vi "ProdaNG.Configurator.Glb.Read.vi"(7 "DB":T2, 8 "error in (no error)":errorcluster) -> (0 "error out":errorcluster, 1 "Configuration":T1={"ShowUnreleased"=TRUE, "Param1"="StepIndex", "ParamStartIdx"=0, "Slots"=1} {"Slots" min=1 max=2; "ParamStartIdx" min=0 max=1}, 2 "Data found":bool)   [LabVIEW 2016]
uses:
  ProdaNG.Configurator.DB.ctl
  ProdaNG.Configurator.Config.ctl
  Tools/Tma.lib/nlconfig.llb/fp2ini mode.ctl
  ProdaNG.Configurator.Glb.vi
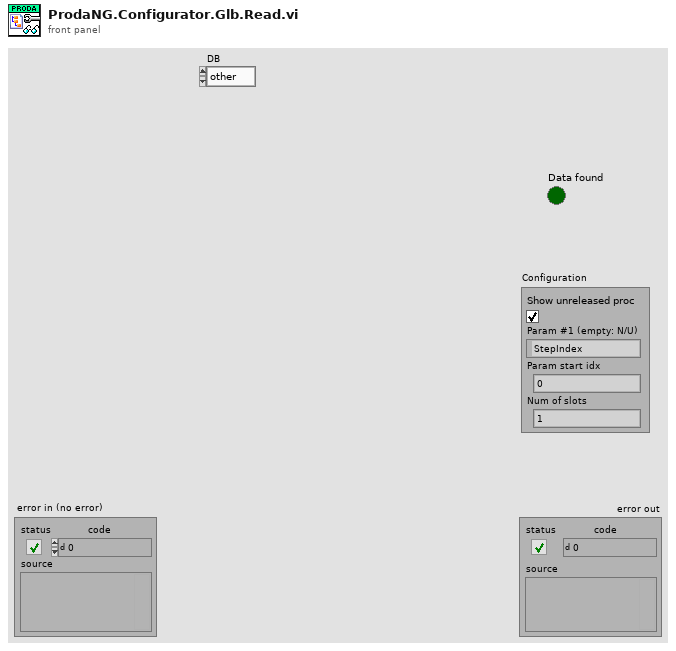
[diagram p1: front panel]
types:
  T1 = typedef "ProdaNG.Configurator.Config.ctl" = cluster{"ShowUnreleased":bool, "Param1":string, "ParamStartIdx":i32, "Slots":i32}
  T2 = typedef "ProdaNG.Configurator.DB.ctl" = enum16{"other", "WPL", "WPK"}
  T3 = typedef "fp2ini mode.ctl" = enum16{"Read Controls", "Write Controls", "Write Indicators", "Read Indicators", "Write all", "Read all"}
  T4 = typedef "ProdaNG.WabcoPart.ctl" = cluster{"i_id":i32, "workCenterId":i32, "contentId":string, "previewId":string, "mdReason":string, "mdUser":string, "mdTime":string, "productName":string, "wabcoNumber":string}
  T5 = typedef "ProdaNG.System.ctl" = cluster{"i_id":i32, "description":string}
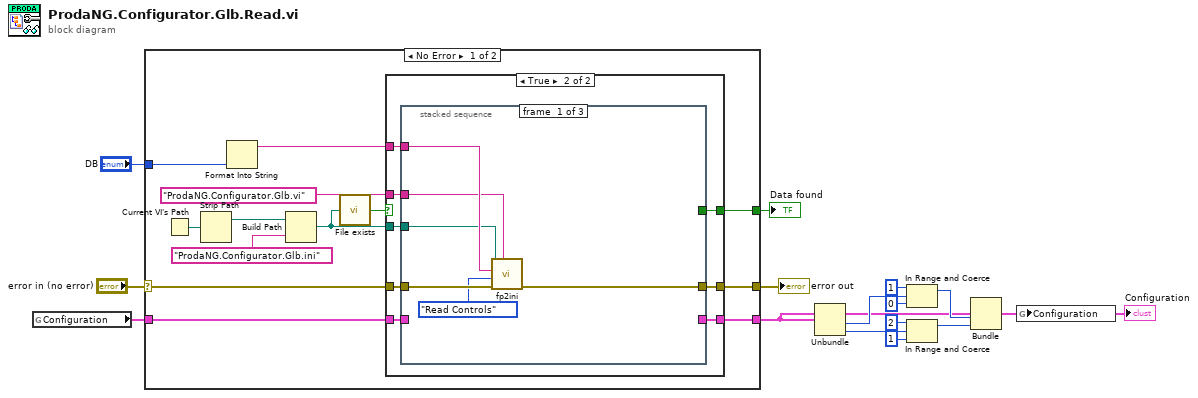
[diagram p0: block diagram]
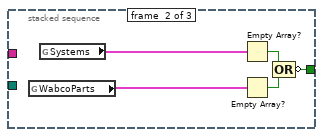
[diagram p3: hidden frame]
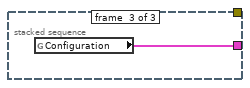
[diagram p4: hidden frame]
diagram:
  n1 = global read "ProdaNG.Configurator.Glb.vi" "Configuration"() -> (w4:T1)
  n2 = case shown="No Error" "error in (no error)" {
    selector: "error in (no error)" -> [w28 w53]
    tunnel: [w27 w53] -> w14
    tunnel: "DB" -> [w22 _]
    tunnel: [w26 _] -> w12
    tunnel: w4 -> [w17 w52]
    tunnel: [w16 w52] -> w3
    frame No Error {
      n3 = Current VI's Path() -> (path=w25:path)
      n4 = Strip Path(path=w25) -> (stripped path=w24:path)  [unwired: 1 out]
      n5 = Format Into String(w22) -> (resulting string=w21:string)  [unwired: 3 in, 1 out]
      n6 = Build Path(base path=w24, name or relative path="ProdaNG.Configurator.Glb.ini") -> (appended path=w19:path)
      n7 = call "File exists.vi"("file path"=w19) -> ("exists?"=w18:bool)  [unwired: 4 in]
      n8 = case shown="True" w18 {
        selector: w18 -> [w30 _]
        tunnel: w28 -> [w31 w39]
        tunnel: [w31 w38] -> w27
        tunnel: [w30 w37] -> w26
        tunnel: w21 -> [_ w36]
        tunnel: "ProdaNG.Configurator.Glb.vi" ("name or relative path") -> [_ w35]
        tunnel: w19 -> [_ w34]
        tunnel: w17 -> [w29 w33]
        tunnel: [w29 w32] -> w16
        frame False {
        }
        frame True {
          n9 = stacked-sequence {
            tunnel: w39 -> [w45 _ _]
            tunnel: [w44 _ _] -> w38
            tunnel: [_ w46 _] -> w37
            tunnel: w36 -> [w42 _ _]
            tunnel: w35 -> [w41 _ _]
            tunnel: w34 -> [w40 _ _]
            tunnel: w33 -> [_ _ _]
            tunnel: [_ _ w51] -> w32
            frame #0 {
              n10 = call "fp2ini.vi"("vi-name (caller if empty)"=w41, "error in"=w45, "mode"=fp2ini_mode."Read Controls", "section"=w42, "ini-file path"=w40) -> ("error out"=w44:errorcluster)  [unwired: 6 in]
            }
            frame #1 {
              n11 = global read "ProdaNG.Configurator.Glb.vi" "WabcoParts"() -> (w49:T4[])
              n12 = global read "ProdaNG.Configurator.Glb.vi" "Systems"() -> (w50:T5[])
              n13 = Empty Array?(array=w50) -> (empty?=w48:bool)
              n14 = Empty Array?(array=w49) -> (empty?=w47:bool)
              n15 = Compound Arithmetic op=OR(w48, w47) -> (invert w46:bool)
            }
            frame #2 {
              n16 = global read "ProdaNG.Configurator.Glb.vi" "Configuration"() -> (w51:T1)
            }
          }
        }
      }
    }
    frame Error {
    }
  }
  "error out" <- w14
  "Data found" <- w12
  n17 = Unbundle(w3) -> ("ParamStartIdx"=w9:i32, "Slots"=w5:i32)  [unwired: 2 out]
  n18 = In Range and Coerce(upper limit=1, x=w9, lower limit=0) -> (coerced(x)=w11:i32)  [unwired: 1 out]
  n19 = In Range and Coerce(upper limit=2, x=w5, lower limit=1) -> (coerced(x)=w6:i32)  [unwired: 1 out]
  n20 = Bundle(cluster=w3, "ParamStartIdx"=w11, "Slots"=w6) -> (w2:T1)  [unwired: 2 in]
  "Configuration" <- w2
  n21 = global write "ProdaNG.Configurator.Glb.vi" "Configuration"(w2) -> ()
